vi "GetText.vi"(8 "error in":errorcluster, 11 "CEF_Serialize node in":refnum<class "CEF_serializable node.lvclass">) -> (0 "error out":errorcluster, 1 "additional text":string, 2 "text":string, 3 "CEF_Serialize node out":refnum<class "CEF_serializable node.lvclass">, 4 "glyph":string)   [LabVIEW 2025, in "CEF.lvlib" / "CEF_serializable node.lvclass"]
doc: "Returns the text representation of the node used for the tree control.Copyright 2017 National Instruments Corporation\n\nLicensed under the Apache License, Version 2.0 (the \"License\"); you may not use this file except in compliance with the License. You may obtain a copy of the License at http://www.apache.org/licenses/LICENSE-2.0\nUnless required by applicable law or agreed to in writing, software distributed under the License is distributed on an \"AS IS\" BASIS, WITHOUT WARRANTIES OR CONDITIONS OF ANY KIND, either express or implied. See the License for the specific language governing permissions and limitations under the License."
uses:
  CEF_serializable node.lvclass
  Node/CEF_Node.lvclass
  serializable configuration/CEF_serializable configuration.lvclass
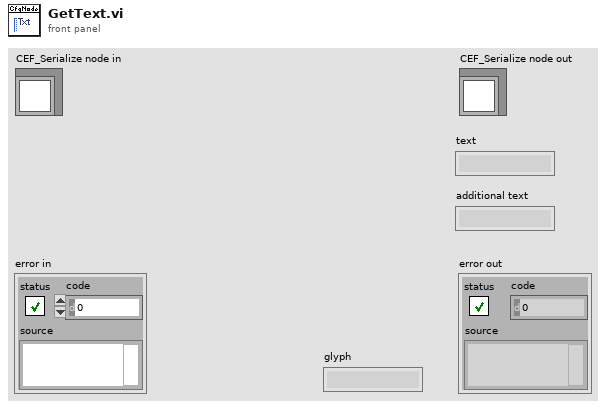
[diagram p1: front panel]
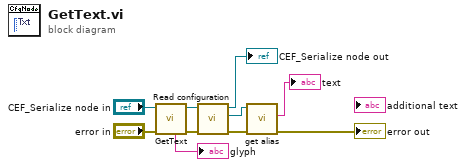
[diagram p0: block diagram]
diagram:
  n1 = call-parent "GetText.vi"("error in"="error in", "CEF_Node in"="CEF_Serialize node in") -> ("error out"=w7:errorcluster, "CEF_Node out"=w6:refnum<class "CEF_serializable node.lvclass">, "glyph"=→"glyph":string)  [unwired: 5 in, 2 out]
  n2 = call-dynamic "Read configuration.vi"("error in"=w7, "CEF_serializable node in"=w6) -> ("error out"=w4:errorcluster, "CEF Configuration"=w3:refnum<class "CEF_serializable configuration.lvclass">, "CEF_serializable node out"=→"CEF_Serialize node out":refnum<class "CEF_serializable node.lvclass">)  [unwired: 7 in]
  n3 = call "get alias.vi"("error in"=w4, "CEF_Configuration in"=w3) -> ("error out"=→"error out":errorcluster, "alias"=→"text":string)  [unwired: 7 in, 1 out]
